vi "calc_PairedPulseWaveform_v0.02.vi"(0 "New input cluster":T1={"Which Position to use for Experiment"=enum."Jumper Safe Position", "Start Position (N)"="", "Jump Position (m)"="", "Duration (s)"=0.0, "Delay (s)"=0.0, "Pulse Width (s)"=0.0, "Replicates"=0.0, "Pulse Delay (s)"=0.0, "Pulse Delta Delay (s)"=0.0, "Vholding (mV)"=0.0, "Valve 1 Position"=1, "Valve 2 Position"=1, "valve 1 used now?"=FALSE, "valve 2 used now?"=FALSE, "valve 3 used now? "=FALSE, "Valve 3 Position"=1, "protocol Preview"=[]} {"Valve 3 Position" min=1 max=8; "Valve 2 Position" min=1 max=8; "Valve 1 Position" min=1 max=8}, 1 "Clear Waveform?":bool, 5 "Old input cluster":T1={"Which Position to use for Experiment"=enum."Jumper Safe Position", "Start Position (N)"="", "Jump Position (m)"="", "Duration (s)"=0.0, "Delay (s)"=0.0, "Pulse Width (s)"=0.0, "Replicates"=0.0, "Pulse Delay (s)"=0.0, "Pulse Delta Delay (s)"=0.0, "Vholding (mV)"=0.0, "Valve 1 Position"=1, "Valve 2 Position"=1, "valve 1 used now?"=FALSE, "valve 2 used now?"=FALSE, "valve 3 used now? "=FALSE, "Valve 3 Position"=1, "protocol Preview"=[]} {"Valve 3 Position" min=1 max=8; "Valve 2 Position" min=1 max=8; "Valve 1 Position" min=1 max=8}, 7 "Numeric":i32=10000, 9 "Jump Filter Freq (Hz)":dbl=30.0, 11 "error in":errorcluster) -> (4 "output cluster":T1={"Which Position to use for Experiment"=enum."Jumper Safe Position", "Start Position (N)"="", "Jump Position (m)"="", "Duration (s)"=0.0, "Delay (s)"=0.0, "Pulse Width (s)"=0.0, "Replicates"=0.0, "Pulse Delay (s)"=0.0, "Pulse Delta Delay (s)"=0.0, "Vholding (mV)"=0.0, "Valve 1 Position"=1, "Valve 2 Position"=1, "valve 1 used now?"=FALSE, "valve 2 used now?"=FALSE, "valve 3 used now? "=FALSE, "Valve 3 Position"=1, "protocol Preview"=[]} {"Valve 3 Position" min=1 max=8; "Valve 2 Position" min=1 max=8; "Valve 1 Position" min=1 max=8}, 15 "error out":errorcluster)   [LabVIEW 2019]
uses:
  <vilib>/Analysis/3filter.llb/Filter Passband Type.ctl
  <vilib>/Analysis/3filter.llb/Bessel Filter (DBL).vi
  <vilib>/measure/NI_MABase.lvlib
  <vilib>/Analysis/NI_AALBase.lvlib
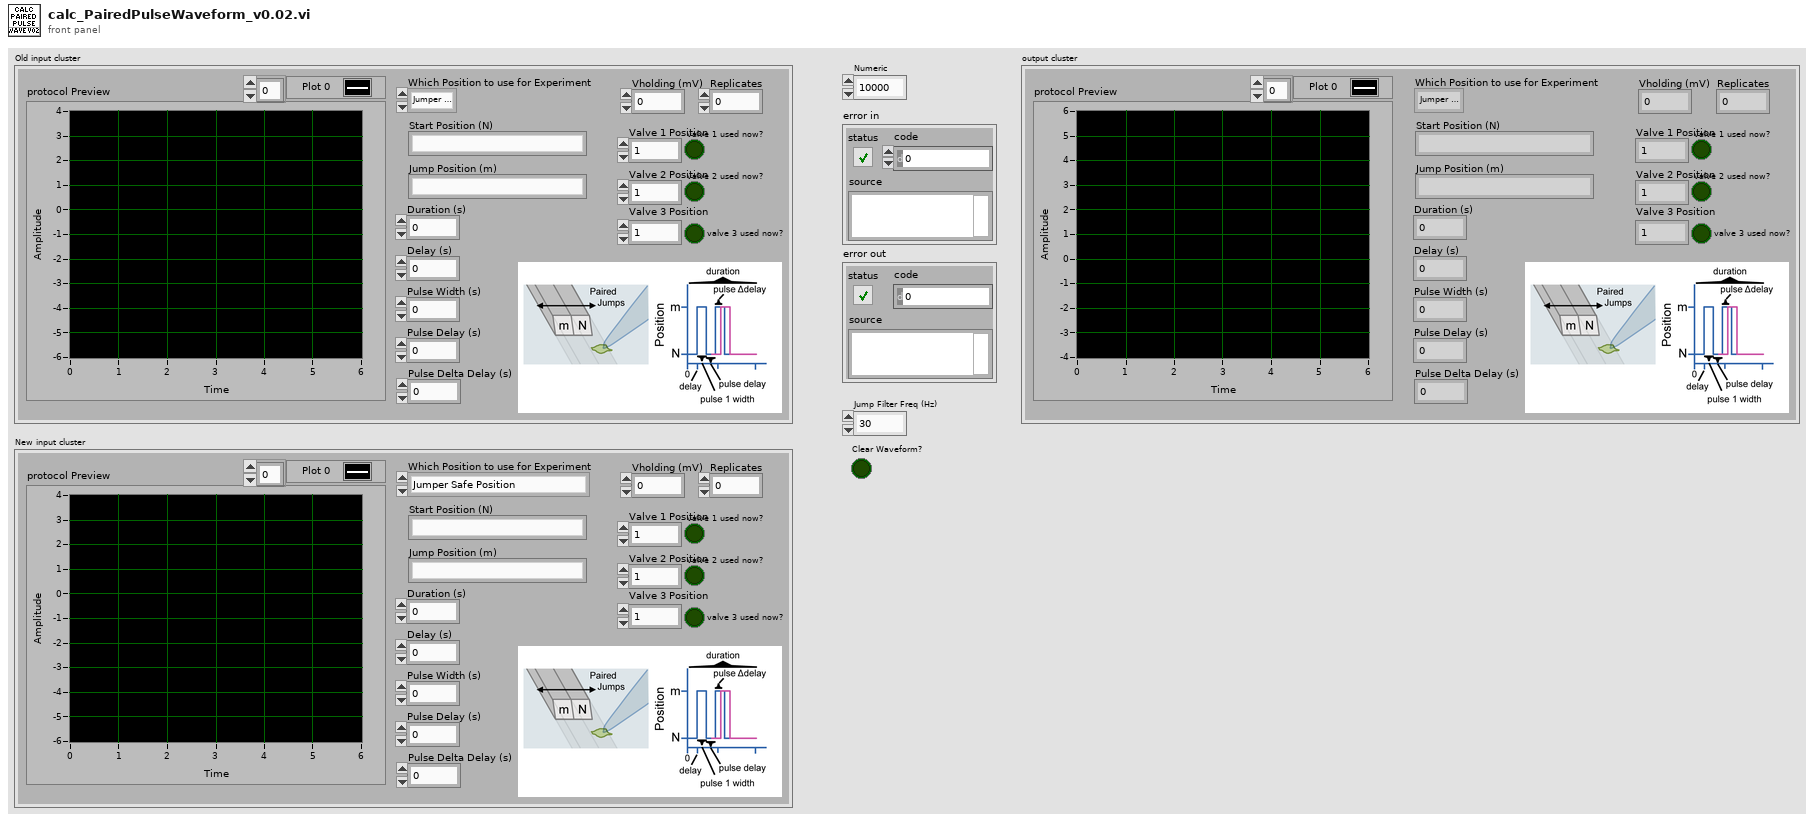
[diagram p1: front panel]
types:
  T1 = cluster{"Which Position to use for Experiment":enum16{"Jumper Safe Position", "Experiment Safe Position", "Jumper Position A", "Jumper Position B", "Jumper Position C", "Jumper Position o-A", "Jumper Position A-o", "Jumper Position A-B", "Jumper Position B-A", "Jumper Position B-C", "Jumper Position C-B", "Jumper Position C-o", "Jumper Position o-C", "Don't Move"}, "Start Position (N)":string, "Jump Position (m)":string, "Duration (s)":dbl, "Delay (s)":dbl, "Pulse Width (s)":dbl, "Replicates":dbl, "Pulse Delay (s)":dbl, "Pulse Delta Delay (s)":dbl, "Vholding (mV)":dbl, "Valve 1 Position":i16, "Valve 2 Position":i16, "valve 1 used now?":bool, "valve 2 used now?":bool, "valve 3 used now? ":bool, "Valve 3 Position":i16, "protocol Preview":waveform(dbl)[]}
  T2 = enum16{"Jumper Safe Position", "Experiment Safe Position", "Jumper Position A", "Jumper Position B", "Jumper Position C", "Jumper Position o-A", "Jumper Position A-o", "Jumper Position A-B", "Jumper Position B-A", "Jumper Position B-C", "Jumper Position C-B", "Jumper Position C-o", "Jumper Position o-C", "Don't Move"}
  T3 = typedef "NI_AALBase.lvlib/Filter Passband Type.ctl" = enum32{"Lowpass", "Highpass", "Bandpass", "Bandstop"}
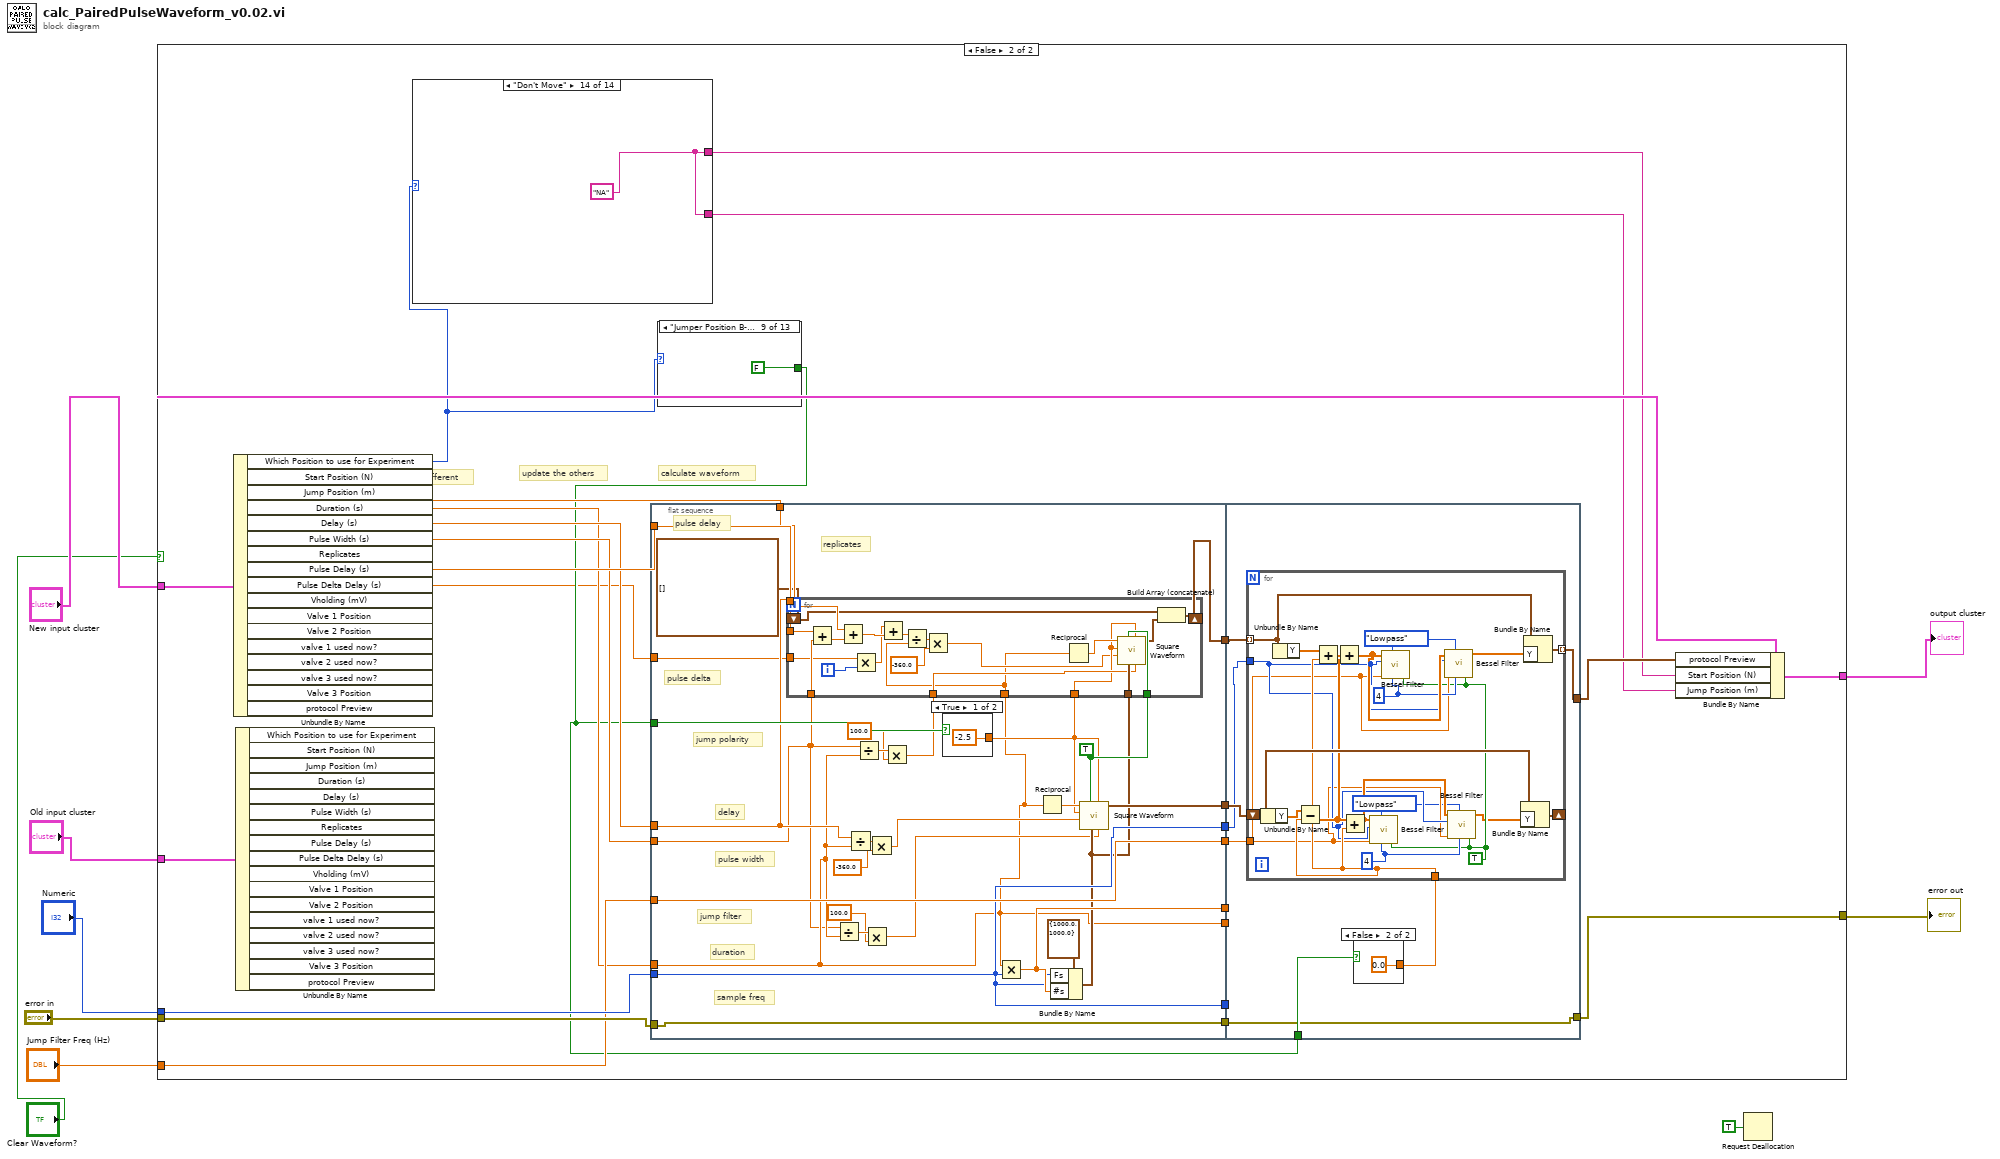
[diagram p0: block diagram]
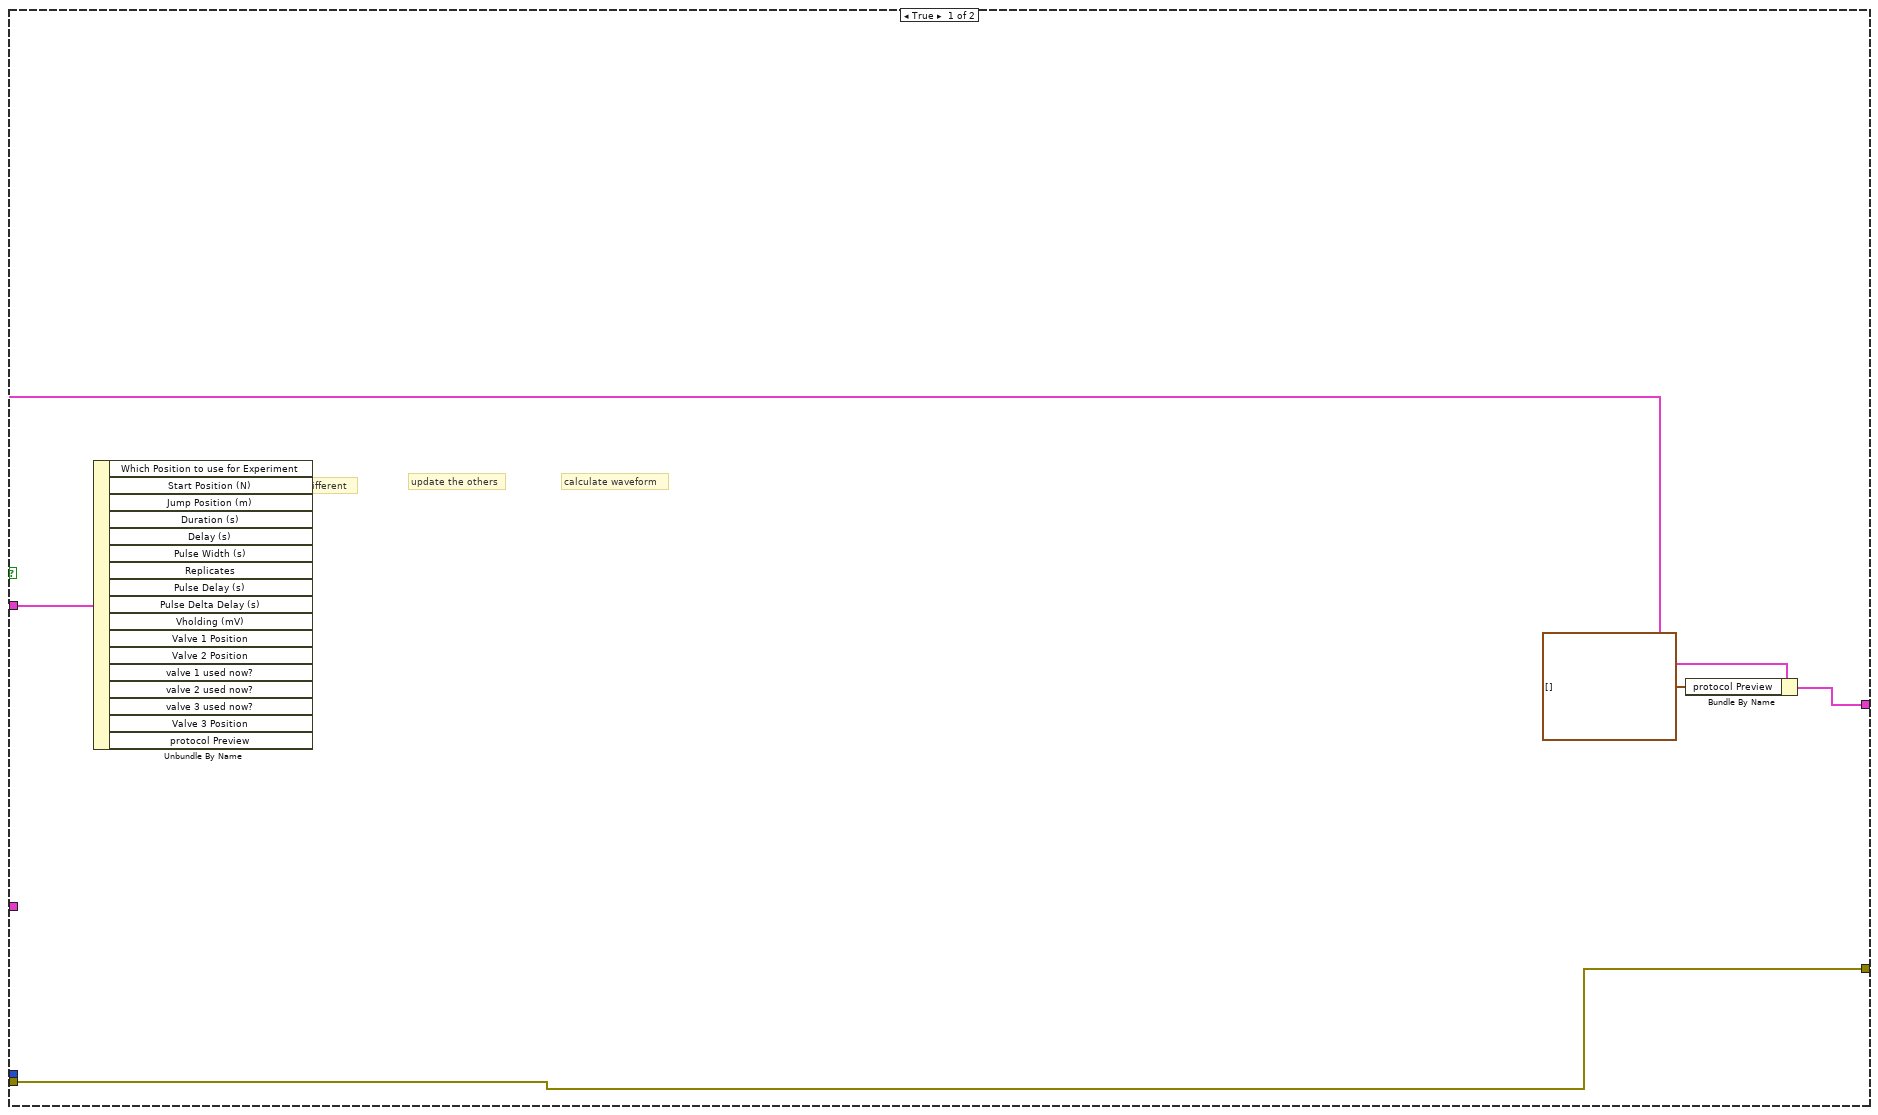
[diagram p2: hidden frame]
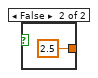
[diagram p3: hidden frame]
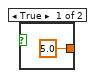
[diagram p4: hidden frame]
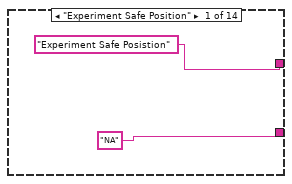
[diagram p5: hidden frame]
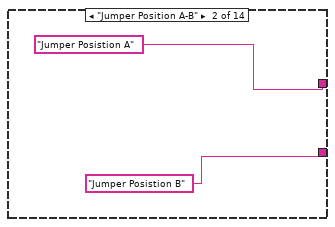
[diagram p6: hidden frame]
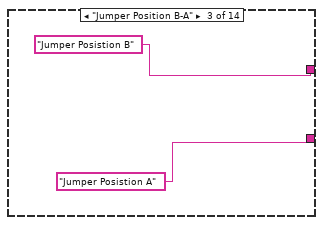
[diagram p7: hidden frame]
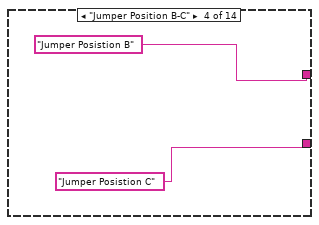
[diagram p8: hidden frame]
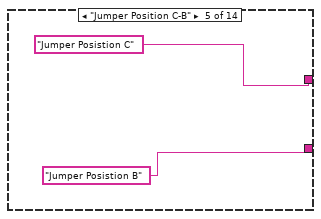
[diagram p9: hidden frame]
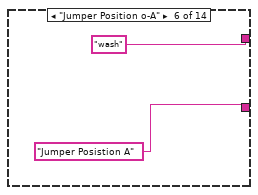
[diagram p10: hidden frame]
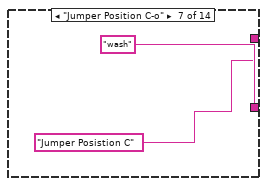
[diagram p11: hidden frame]
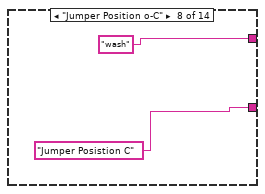
[diagram p12: hidden frame]
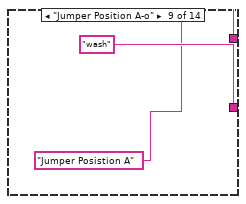
[diagram p13: hidden frame]
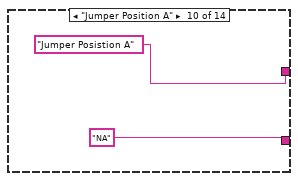
[diagram p14: hidden frame]
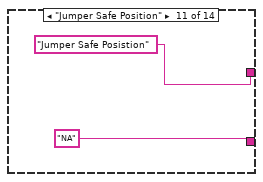
[diagram p15: hidden frame]
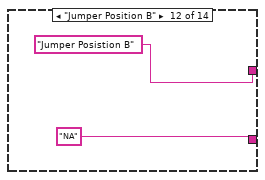
[diagram p16: hidden frame]
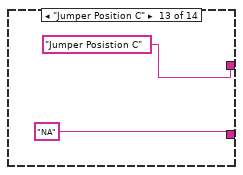
[diagram p17: hidden frame]
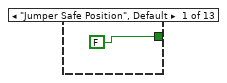
[diagram p18: hidden frame]
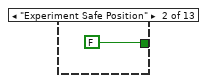
[diagram p19: hidden frame]
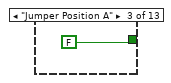
[diagram p20: hidden frame]
diagram:
  n1 = case shown="False" "Clear Waveform?" {
    tunnel: "New input cluster" -> [w13 w31]
    tunnel: [w12 w30] -> w8
    tunnel: "Old input cluster" -> [_ w29]
    tunnel: "Numeric" -> [_ w28]
    tunnel: "error in" -> [w11 w27]
    tunnel: "Jump Filter Freq (Hz)" -> [_ w23]
    tunnel: [w11 w19] -> w3
    frame True {
      # "calculate waveform"
      # "update the others"
      # "which is different"
      n2 = Unbundle By Name(w13) -> ()  [unwired: 17 out]
      n3 = Bundle By Name(cluster=w13, "protocol Preview"=waveform(dbl)[] []) -> (w12:T1)
    }
    frame False {
      # "calculate waveform"
      # "update the others"
      # "which is different"
      n4 = Unbundle By Name(w31) -> ("Which Position to use for Experiment"=w16:T2, "Duration (s)"=w22:dbl, "Delay (s)"=w25:dbl, "Pulse Width (s)"=w24:dbl, "Replicates"=w21:dbl, "Pulse Delay (s)"=w26:dbl, "Pulse Delta Delay (s)"=w17:dbl)  [unwired: 10 out]
      n5 = Unbundle By Name(w29) -> ()  [unwired: 17 out]
      n6 = case shown="\"Don't Move\"" w16 {
        tunnel: ["Experiment Safe Posistion" "Jumper Posistion A" "Jumper Posistion B" "Jumper Posistion B" "Jumper Posistion C" "wash" "Jumper Posistion C" "wash" "Jumper Posistion A" "Jumper Posistion A" "Jumper Safe Posistion" "Jumper Posistion B" "Jumper Posistion C" w147] -> w15
        tunnel: ["NA" "Jumper Posistion B" "Jumper Posistion A" "Jumper Posistion C" "Jumper Posistion B" "Jumper Posistion A" "wash" "Jumper Posistion C" "wash" "NA" "NA" "NA" "NA" w147] -> w14
        frame "Experiment Safe Position" {
        }
        frame "Jumper Position A-B" {
        }
        frame "Jumper Position B-A" {
        }
        frame "Jumper Position B-C" {
        }
        frame "Jumper Position C-B" {
        }
        frame "Jumper Position o-A" {
        }
        frame "Jumper Position C-o" {
        }
        frame "Jumper Position o-C" {
        }
        frame "Jumper Position A-o" {
        }
        frame "Jumper Position A" {
        }
        frame "Jumper Safe Position" {
        }
        frame "Jumper Position B" {
        }
        frame "Jumper Position C" {
        }
        frame "Don't Move" {
          w147 = "NA"
        }
      }
      n7 = flat-sequence {
        tunnel: w22 -> [w42]
        tunnel: w23 -> [w65]
        tunnel: w28 -> [w64]
        tunnel: [w66] -> w39
        tunnel: [w64] -> w38
        tunnel: [w65] -> w37
        tunnel: [w64] -> w36
        tunnel: [w63] -> w35
        tunnel: w27 -> [w62]
        tunnel: [w62] -> w34
        tunnel: w18 -> [w61]
        tunnel: [w42] -> w33
        tunnel: w25 -> [w46]
        tunnel: w24 -> [w41]
        tunnel: [w51] -> w32
        tunnel: w26 -> [w45]
        tunnel: w21 -> [w44]
        tunnel: w17 -> [w43]
        tunnel: w39 -> [_]
        tunnel: w38 -> [_]
        tunnel: w37 -> [w95]
        tunnel: w36 -> [w96]
        tunnel: w35 -> [w98]
        tunnel: w34 -> [w91]
        tunnel: w18 -> [w97]
        tunnel: w33 -> [_]
        tunnel: w32 -> [w93]
        tunnel: [w92] -> w20
        tunnel: [w91] -> w19
        frame #0 {
          w55 = TRUE ("reset signal")
          # "replicates"
          # "sample freq"
          # "duration"
          # "jump filter"
          # "pulse width"
          # "delay"
          # "jump polarity"
          # "pulse delta"
          # "pulse delay"
          n8 = Divide(x=w41, y=w42) -> (x/y=w60:dbl)
          n9 = Divide(x=w46, y=w42) -> (x/y=w57:dbl)
          n10 = Divide(x=w41, y=w42) -> (x/y=w53:dbl)
          n11 = Multiply(x=w60, y=100.0) -> (x*y=w49:dbl)
          n12 = Multiply(x=w57, y=-360.0) -> (x*y=w54:dbl)
          n13 = Multiply(x=w53, y=100.0) -> (x*y=w48:dbl)
          n14 = case shown="True" w61 {
            tunnel: [-2.5 ("Amplitude") 2.5 ("Amplitude")] -> w47
            frame True {
            }
            frame False {
            }
          }
          n15 = Multiply(x=w42, y=w64) -> (x*y=w66:dbl)
          n16 = Reciprocal(x=w42) -> (1/x=w56:dbl)
          n17 = Bundle By Name(cluster=cluster{"Fs":dbl, "#s":dbl} {"Fs"=1000.0, "#s"=1000.0} ("sampling info"), "Fs"=w64, "#s"=w66) -> (w50:cluster{"Fs":dbl, "#s":dbl})
          n18 = for {
            N: w44 -> [_]
            tunnel: w55 -> [w88]
            tunnel: w50 -> [w87]
            tunnel: w48 -> [w85]
            tunnel: w47 -> [w84]
            tunnel: w41 -> [w79]
            tunnel: w46 -> [w78]
            tunnel: w45 -> [w77]
            tunnel: w42 -> [w75]
            shift-right: [w73] -> w51
            shift-left: waveform(dbl)[] [] -> [w72]
            tunnel: w43 -> [w68]
            i -> [w70]
            n19 = Add(x=w78, y=w79) -> (x+y=w82:dbl)
            n20 = Add(x=w77, y=w82) -> (x+y=w83:dbl)
            n21 = Multiply(x=w68, y=w70) -> (x*y=w69:dbl)
            n22 = Add(x=w69, y=w83) -> (x+y=w71:dbl)
            n23 = Divide(x=w71, y=w75) -> (x/y=w81:dbl)
            n24 = Multiply(x=w81, y=-360.0) -> (x*y=w80:dbl)
            n25 = Reciprocal(x=w75) -> (1/x=w86:dbl)
            n26 = call <vilib>:"Square Waveform.vi"("duty cycle (%)"=w85, "offset"=w84, "sampling info"=w87, "reset signal"=w88, "phase"=w80, "amplitude"=w84, "frequency"=w86) -> ("signal out"=w74:waveform(dbl))  [unwired: 3 in, 1 out]
            n27 = Build Array (concatenate)(w72, w74) -> (w73:waveform(dbl)[])
          }
          n28 = call <vilib>:"Square Waveform.vi"("duty cycle (%)"=w49, "offset"=w47, "sampling info"=w50, "reset signal"=w55, "phase"=w54, "amplitude"=w47, "frequency"=w56) -> ("signal out"=w63:waveform(dbl))  [unwired: 3 in, 1 out]
        }
        frame #1 {
          n29 = case shown="False" w97 {
            tunnel: [5.0 ("Amplitude") 0.0 ("Amplitude")] -> w94
            frame True {
            }
            frame False {
            }
          }
          n30 = for {
            tunnel: w96 -> [w104]
            tunnel: w95 -> [w103]
            tunnel: w94 -> [w106]
            tunnel: w93 -> [w116] mode=indexing
            shift-right: [w118] -> _
            shift-left: w98 -> [w117]
            tunnel: [w115] -> w92 mode=indexing
            w100 = TRUE ("init/cont (init:F)")
            w108 = 4 ("order")
            w107 = Filter_Passband_Type."Lowpass" ("filter type")
            w101 = 4 ("order")
            w102 = Filter_Passband_Type."Lowpass" ("filter type")
            n31 = Unbundle By Name(w117) -> ("Y"=w114:dbl[])
            n32 = Unbundle By Name(w116) -> ("Y"=w113:dbl[])
            n33 = Subtract(x=w114, y=w106) -> (x-y=w111:dbl[])
            n34 = Add(x=w113, y=w106) -> (x+y=w112:dbl[])
            n35 = Add(x=w112, y=w111) -> (x+y=w110:dbl[])
            n36 = Add(x=w111, y=w106) -> (x+y=w105:dbl[])
            n37 = call-poly <vilib>:"Bessel Filter.vi"("init/cont (init:F)"=w100, "order"=w101, "filter type"=w102, "low cutoff freq: fl"=w103, "sampling freq: fs"=w104, "X"=w105) -> ()  [unwired: 2 in, 2 out]
            n38 = call-poly <vilib>:"Bessel Filter.vi"("init/cont (init:F)"=w100, "order"=w108, "filter type"=w107, "low cutoff freq: fl"=w103, "sampling freq: fs"=w104, "X"=w110) -> ()  [unwired: 2 in, 2 out]
            n39 = call-poly <vilib>:"Bessel Filter.vi"("init/cont (init:F)"=w100, "order"=w108, "filter type"=w107, "low cutoff freq: fl"=w103, "sampling freq: fs"=w104, "X"=w110) -> ("Filtered X"=w109:dbl[])  [unwired: 2 in, 1 out]
            n40 = call-poly <vilib>:"Bessel Filter.vi"("init/cont (init:F)"=w100, "order"=w101, "filter type"=w102, "low cutoff freq: fl"=w103, "sampling freq: fs"=w104, "X"=w105) -> ("Filtered X"=w99:dbl[])  [unwired: 2 in, 1 out]
            n41 = Bundle By Name(cluster=w117, "Y"=w99) -> (w118:waveform(dbl))
            n42 = Bundle By Name(cluster=w116, "Y"=w109) -> (w115:waveform(dbl))
          }
        }
      }
      n43 = case shown="\"Jumper Position B-A\"" w16 {
        tunnel: [FALSE FALSE FALSE FALSE FALSE TRUE FALSE TRUE FALSE TRUE FALSE TRUE FALSE] -> w18
        frame "Jumper Safe Position", Default {
        }
        frame "Experiment Safe Position" {
        }
        frame "Jumper Position A" {
        }
        frame "Jumper Position B" {
        }
        frame "Jumper Position C" {
        }
        frame "Jumper Position o-A" {
        }
        frame "Jumper Position A-o" {
        }
        frame "Jumper Position A-B" {
        }
        frame "Jumper Position B-A" {
        }
        frame "Jumper Position B-C" {
        }
        frame "Jumper Position C-B" {
        }
        frame "Jumper Position C-o" {
        }
        frame "Jumper Position o-C" {
        }
      }
      n44 = Bundle By Name(cluster=w31, "protocol Preview"=w20, "Start Position (N)"=w15, "Jump Position (m)"=w14) -> (w30:T1)
    }
  }
  "output cluster" <- w8
  "error out" <- w3
  n45 = Request Deallocation(TRUE ("flag")) -> ()
